vi "SetSystemDefinitionPropertyValue_Double.vi"(8 "error in (no error)":errorcluster, 9 "value":dbl, 10 "property name":string, 11 "BaseNodeType in":refnum<k39>) -> (0 "error out":errorcluster, 3 "BaseNodeType out":refnum<k39>)   [LabVIEW 2027, in "VeriStandTestUtilities.lvlib"]
uses:
  VeriStandTestUtilities.lvlib
  C:/NetCoreDLL/NationalInstruments.VeriStand.SystemStorage.dll
  NetCoreDLL/NationalInstruments.VeriStand.SystemStorage.dll
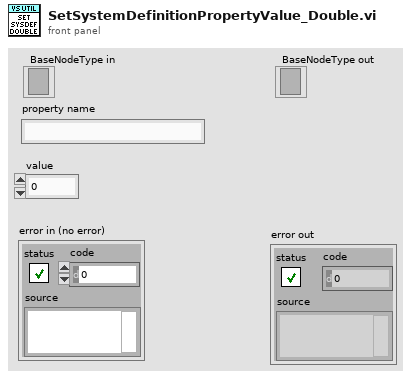
[diagram p1: front panel]
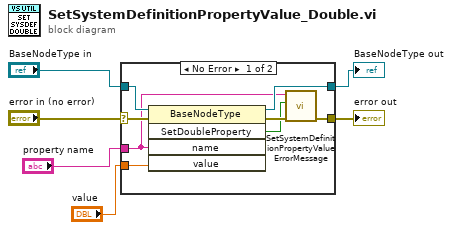
[diagram p0: block diagram]
diagram:
  n1 = case shown="No Error" "error in (no error)" {
    selector: "error in (no error)" -> [w13 w16]
    tunnel: "BaseNodeType in" -> [w14 w15]
    tunnel: "value" -> [w12 _]
    tunnel: "property name" -> [w7 _]
    tunnel: [w11 w15] -> w2
    tunnel: [w9 w16] -> w1
    frame No Error {
      n2 = invoke class="BaseNodeType" method="SetDoubleProperty"(reference=w14, error in=w13, "name"=w7, "value"=w12) -> (reference out=w11:refnum<k39>, error out=w10:errorcluster, "SetDoubleProperty"=w8:bool)  [unwired: 1 in, 2 out]
      n3 = call "SetSystemDefinitionPropertyValueErrorMessage.vi"("error in (no error)"=w10, "successful?"=w8, "property name"=w7) -> ("error out"=w9:errorcluster)  [unwired: 8 in]
    }
    frame Error {
    }
  }
  "error out" <- w1
  "BaseNodeType out" <- w2
